vi "Wait for Disconnect.vi"(8 "error in (no error)":errorcluster, 11 "Websocket Client in":refnum<class "Websocket Client.lvclass">) -> (0 "error out":errorcluster, 3 "Websocket Client out":refnum<class "Websocket Client.lvclass">)   [LabVIEW 2020, in "Stream-Websocket.lvlib" / "Websocket Client.lvclass"]
uses:
  Websocket Client.lvclass
  C:/dev/lv20CE/relink/lv-stream/stream/Connection/Connection.lvclass
  lv-stream/stream/Connection/State.ctl
  Client Command.ctl
  Stream-Websocket.lvlib
  lv-stream/stream/Connection/Connection.lvclass
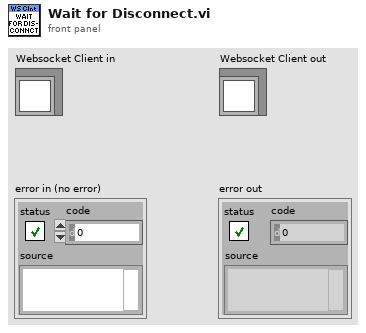
[diagram p1: front panel]
types:
  T1 = typedef "Stream.lvlib/Connection.lvclass/State.ctl" = enum16{"Closed", "Idle", "Connecting", "Connected", "Shutdown"}
  T2 = typedef "Stream-Websocket.lvlib/Client Command.ctl" = enum16{"Connect", "Close", "Shutdown", "Reconnect"}
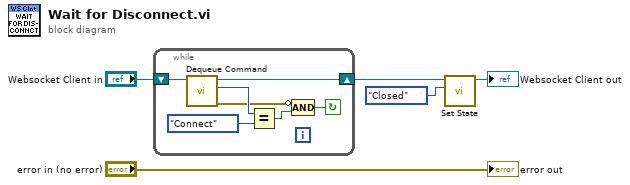
[diagram p0: block diagram]
diagram:
  n1 = while {
    shift-right: [w6] -> w2
    shift-left: "Websocket Client in" -> [w12]
    stop <- w7 continue-if-true
    n2 = call "Dequeue Command.vi"("Websocket Client in"=w12) -> ("error out"=w9:errorcluster, "Command"=w11:T2, "Websocket Client out"=w6:refnum<class "Websocket Client.lvclass">)  [unwired: 7 in, 1 out]
    n3 = Equal?(x=w11, y=Client_Command."Connect") -> (x = y?=w8:bool)
    n4 = Compound Arithmetic op=AND(invert w9, w8) -> (w7:bool)
  }
  n5 = call "Set State.vi"("State"=State."Closed", "Connection in"=w2) -> ("Connection out"=→"Websocket Client out":refnum<class "Websocket Client.lvclass">)  [unwired: 8 in, 1 out]
  "error out" <- "error in (no error)"
